vi "Get Legend Label Property.vi"(8 "error in (no error)":errorcluster, 9 "Active Axis":enum16{"X-axis", "Y-axis", "Z-axis"}(ring)=enum."Z-axis", 10 "Plot Range":T1, 11 "3D Plot in":refnum<class "3D Plot.lvclass">) -> (0 "error out":errorcluster, 1 "Range Min":sgl, 2 "Range Max":sgl, 3 "3D Plot out":refnum<class "3D Plot.lvclass">)   [LabVIEW 2020, in "3D Plot.lvclass"]
uses:
  3D Plot.lvclass
  Range Clusters.ctl
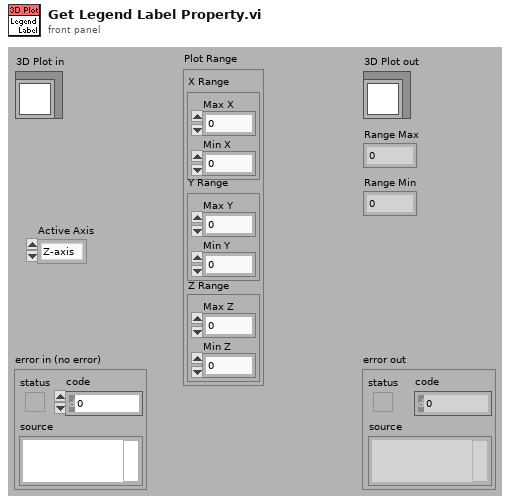
[diagram p1: front panel]
types:
  T1 = typedef "3D Plot.lvclass/Range Clusters.ctl" = cluster{"X Range":cluster{"Max X":sgl, "Min X":sgl}, "Y Range":cluster{"Max Y":sgl, "Min Y":sgl}, "Z Range":cluster{"Max Z":sgl, "Min Z":sgl}}
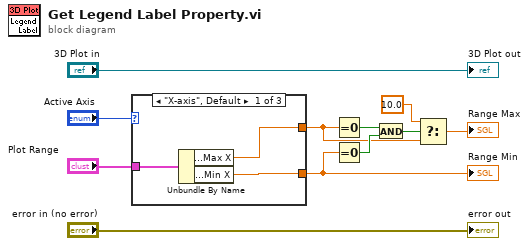
[diagram p0: block diagram]
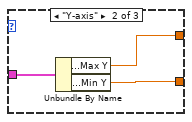
[diagram p2: hidden frame]
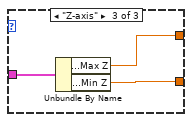
[diagram p3: hidden frame]
diagram:
  n1 = case shown="\"X-axis\", Default" "Active Axis" {
    tunnel: "Plot Range" -> [w12 w15 w20]
    tunnel: [w14 w17 w19] -> w2
    tunnel: [w13 w16 w18] -> w7
    frame "X-axis", Default {
      n2 = Unbundle By Name(w12) -> ("X Range.Max X"=w14:sgl, "X Range.Min X"=w13:sgl)
    }
    frame "Y-axis" {
      n3 = Unbundle By Name(w15) -> ("Y Range.Max Y"=w17:sgl, "Y Range.Min Y"=w16:sgl)
    }
    frame "Z-axis" {
      n4 = Unbundle By Name(w20) -> ("Z Range.Max Z"=w19:sgl, "Z Range.Min Z"=w18:sgl)
    }
  }
  "Range Min" <- w7
  n5 = Equal To 0?(x=w2) -> (x = 0?=w6:bool)
  n6 = Equal To 0?(x=w7) -> (x = 0?=w5:bool)
  n7 = And(x=w6, y=w5) -> (x .and. y?=w3:bool)
  n8 = Select(t=sgl 10.0, s=w3, f=w2) -> (s? t:f=→"Range Max":sgl)
  "3D Plot out" <- "3D Plot in"
  "error out" <- "error in (no error)"
